vi "Test Sinewave Module.vi"(8 "error in":errorcluster, 11 "TestCase in":refnum<class "Test FGEN.lvclass">) -> (0 "error out":errorcluster, 3 "TestCase out":refnum<class "Test FGEN.lvclass">)   [LabVIEW 2020, in "Test FGEN.lvclass"]
uses:
  Test FGEN.lvclass
  <vilib>/addons/_JKI Toolkits/VI Tester/TestCase.llb/TestCase.lvclass
  Libraries/FGen/FGen.lvlib
  <vilib>/measure/NI_MABase.lvlib
  C:/Program Files (x86)/National Instruments/LabVIEW 2020/vi.lib/addons/_JKI Toolkits/VI Tester/TestCase.llb/TestCase.lvclass
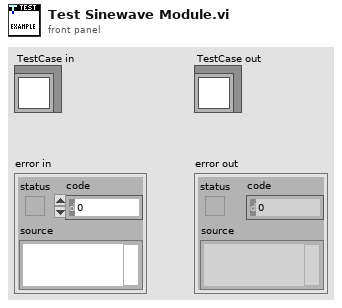
[diagram p1: front panel]
types:
  T1 = enum16{"Sine Wave", "Triangle Wave", "Square Wave", "Sawtooth Wave"}
  T2 = typedef "FGen.lvlib/Generate Signal (Reply Payload)--cluster.ctl" = cluster{"signal out":waveform(dbl), "Generate Signal_error":errorcluster}
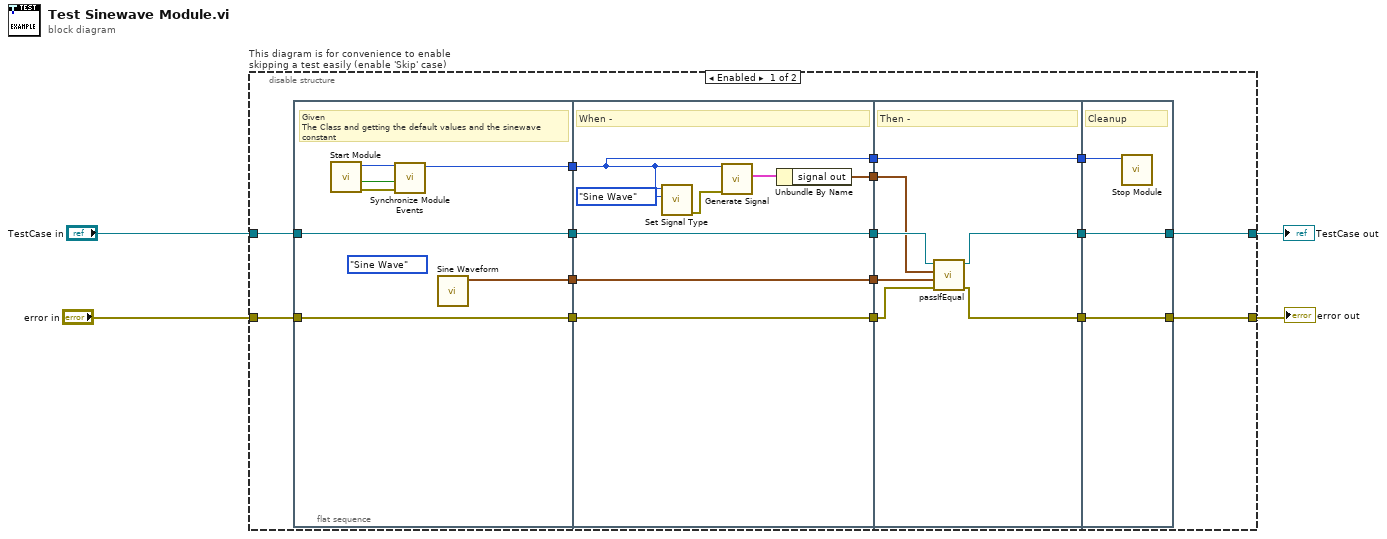
[diagram p0: block diagram]
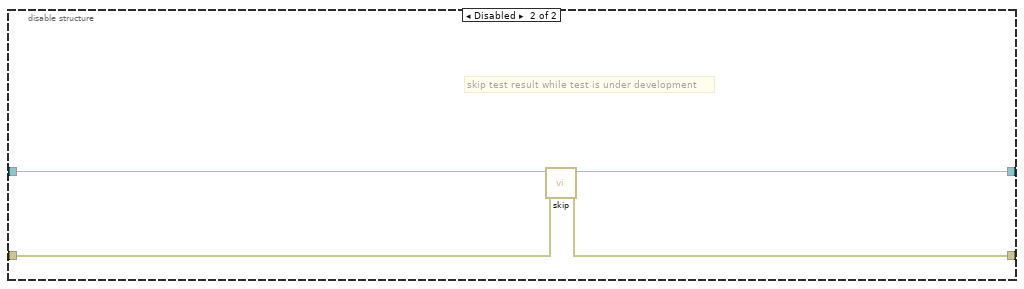
[diagram p2: hidden frame]
diagram:
  n1 = disable-structure "This diagram is for convenience to enable skipping a test easily (enable 'Skip' case)" shown="Enabled" {
    disable-tunnel: "TestCase in" -> [w12 w47]
    disable-tunnel: [w11 w46] -> w1
    disable-tunnel: [w19 w49] -> w3
    disable-tunnel: "error in" -> [w18 w48]
    frame Enabled {
      n2 = flat-sequence {
        tunnel: w12 -> [w25]
        tunnel: [w25] -> w15
        tunnel: w18 -> [w27]
        tunnel: [w27] -> w16
        tunnel: [w21] -> w9
        tunnel: [w23] -> w8
        tunnel: [w34] -> w14
        tunnel: w15 -> [w34]
        tunnel: [w35] -> w17
        tunnel: w16 -> [w35]
        tunnel: [w33] -> w10
        tunnel: w9 -> [w33]
        tunnel: w8 -> [w29]
        tunnel: [w31] -> w7
        tunnel: [w29] -> w6
        tunnel: [w39] -> w13
        tunnel: [w42] -> w20
        tunnel: w14 -> [w40]
        tunnel: w17 -> [w41]
        tunnel: w10 -> [w38]
        tunnel: w7 -> [w37]
        tunnel: w6 -> [w36]
        tunnel: [w36] -> w5
        tunnel: [w45] -> w19
        tunnel: [w44] -> w11
        tunnel: w13 -> [w44]
        tunnel: w20 -> [w45]
        tunnel: w5 -> [w43]
        frame #0 {
          (unwired) T1."Sine Wave" ("signal type")
          # "Given\nThe Class and getting the default values and the sinewave constant"
          n3 = call "Start Module.vi"() -> ("error out"=w26:errorcluster, "Wait for Event Sync?"=w22:bool, "Module ID"=w24:i32)  [unwired: 8 in, 1 out]
          n4 = call "Synchronize Module Events.vi"("error in"=w26, "Wait for Event Sync?"=w22, "Module ID in"=w24) -> ("Module ID out"=w23:i32)  [unwired: 7 in, 1 out]
          n5 = call <vilib>:"Sine Waveform.vi"() -> ("signal out"=w21:waveform(dbl))  [unwired: 10 in, 1 out]
        }
        frame #1 {
          # "When -"
          n6 = call "Set Signal Type.vi"("signal type"=T1."Sine Wave", "Module ID"=w29) -> ("error out"=w30:errorcluster)  [unwired: 9 in]
          n7 = call "Generate Signal.vi"("error in"=w30, "Module ID"=w29) -> ("Reply Payload"=w32:T2)  [unwired: 7 in, 2 out]
          n8 = Unbundle By Name(w32) -> ("signal out"=w31:waveform(dbl))
        }
        frame #2 {
          # "Then -"
          n9 = call-dynamic "passIfEqual.vi"("error in (no error)"=w41, "y"=w38, "x"=w37, "TestCase in"=w40) -> ("error out"=w42:errorcluster, "TestCase out"=w39:refnum<class "Test FGEN.lvclass">)  [unwired: 6 in]
        }
        frame #3 {
          # "Cleanup"
          n10 = call "Stop Module.vi"("Module ID"=w43) -> ()  [unwired: 10 in, 1 out]
        }
      }
    }
    frame Disabled {
      # "skip test result while test is under development"
      n11 = call <vilib>:"skip.vi"("error in (no error)"=w48, "TestCase in"=w47) -> ("error out"=w49:errorcluster, "TestCase out"=w46:refnum<class "Test FGEN.lvclass">)  [unwired: 8 in]
    }
  }
  "error out" <- w3
  "TestCase out" <- w1
